vi "TCP MC Client_2.vi"() -> ()   [LabVIEW 2018]
panel:
  out "에러 출력":errorcluster
  out "웨이브폼 차트":i32(graph)
  in  "정지":bool
  in  "주소":string
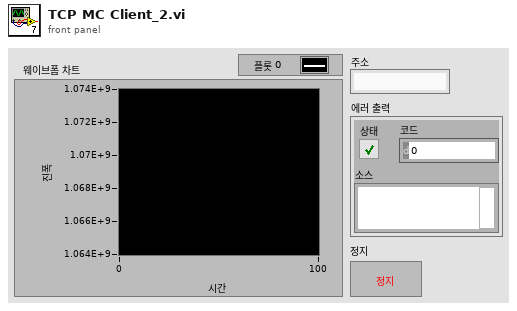
[diagram p1: front panel]
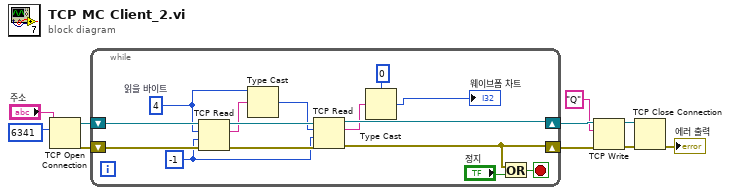
[diagram p0: block diagram]
diagram:
  n1 = TCP Open Connection(address="주소", remote port or service name=u16 6341 ("원격 포트 또는 서비스 이름")) -> (connection ID=w10:refnum<k5>, error out=w9:errorcluster)  [unwired: 3 in]
  n2 = while {
    shift-right: [w18] -> w3
    shift-left: w10 -> [w20]
    shift-right: [w22] -> w2
    shift-left: w9 -> [w25]
    stop <- w21 stop-if-true
    w14 = -1 ("타임아웃 ms (25000)")
    w16 = 4  # 읽을 바이트
    n3 = TCP Read(connection ID=w20, bytes to read=w16, error in (no error)=w25, 9:w14) -> (connection ID out=w19:refnum<k5>, data out=w17:string, error out=w24:errorcluster)  [unwired: 1 in]
    n4 = Type Cast(type=w16, x=w17) -> (*(type *) &x=w15:i32)
    n5 = TCP Read(connection ID=w19, bytes to read=w15, error in (no error)=w24, 9:w14) -> (connection ID out=w18:refnum<k5>, data out=w13:string, error out=w22:errorcluster)  [unwired: 1 in]
    n6 = Type Cast(type=0, x=w13) -> (*(type *) &x=→"웨이브폼 차트":i32)
    n7 = Or(x=w22, y="정지") -> (x .or. y?=w21:bool)
  }
  n8 = TCP Write(connection ID=w3, data in="Q" ("데이터 입력"), error in (no error)=w2) -> (connection ID out=w5:refnum<k5>, error out=w6:errorcluster)  [unwired: 1 in, 1 out]
  n9 = TCP Close Connection(connection ID=w5, error in (no error)=w6) -> (error out=→"에러 출력":errorcluster)  [unwired: 1 in, 1 out]
